vi "Processing_Dequeue.vi"(4 "Offset (0) / 1E-5":dbl, 6 "Amp (1E6) / V A-1":dbl=1000000.0, 11 "Flushed Elements":cluster{"Array":dbl[][]}[](array[cluster])) -> (1 "G / G0":dbl[](array[numeric]), 2 "Bias / V":dbl[](array[numeric]), 3 "Piezo / nm":dbl[](array[numeric]), 5 "Femto / V":dbl[](array[numeric]))   [LabVIEW 2025]
panel:
  in  "Piezo Sensitivity / nm V-1":dbl=1.95
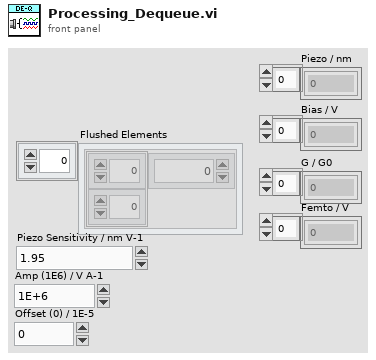
[diagram p1: front panel]
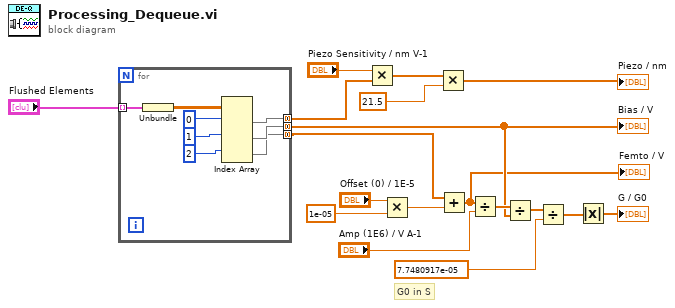
[diagram p0: block diagram]
diagram:
  # "G0 in S"
  n1 = for {
    tunnel: "Flushed Elements" -> [w26] mode=indexing
    tunnel: [w21] -> w16 mode=concatenating
    tunnel: [w20] -> w9 mode=concatenating
    tunnel: [w19] -> w12 mode=concatenating
    n2 = Unbundle(w26) -> ("Array"=w25:dbl[][])
    n3 = Index Array(array=w25, index (row) #1=0 ("index"), index (row) #2=1 ("index"), index (row) #3=2 ("index")) -> (element #1=w21:dbl[], element #2=w20:dbl[], element #3=w19:dbl[])  [unwired: 3 in]
  }
  "Bias / V" <- w9
  n4 = Multiply(x="Piezo Sensitivity / nm V-1", y=w16) -> (x*y=w2:dbl[])
  n5 = Multiply(x="Offset (0) / 1E-5", y=1e-05) -> (x*y=w13:dbl)
  n6 = Multiply(x=w2, y=21.5) -> (x*y=→"Piezo / nm":dbl[])
  n7 = Add(x=w12, y=w13) -> (x+y=w4:dbl[])
  "Femto / V" <- w4
  n8 = Divide(x=w4, y="Amp (1E6) / V A-1") -> (x/y=w10:dbl[])
  n9 = Divide(x=w10, y=w9) -> (x/y=w8:dbl[])
  n10 = Divide(x=w8, y=7.7480917e-05) -> (x/y=w6:dbl[])
  n11 = Absolute Value(x=w6) -> (abs(x)=→"G / G0":dbl[])
